vi "Default User.vi"(1 "Account in":string) -> (0 "Account out":string)   [LabVIEW 2019, in "SelfUpdate.lvclass"]
uses:
  SelfUpdate.lvclass
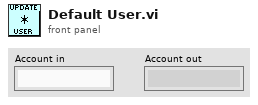
[diagram p1: front panel]
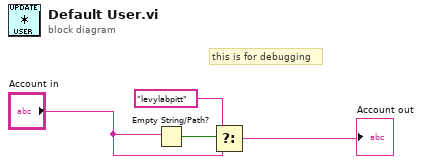
[diagram p0: block diagram]
diagram:
  # "this is for debugging"
  n1 = Empty String/Path?(string/path="Account in") -> (empty?=w1:bool)
  n2 = Select(t="levylabpitt", s=w1, f="Account in") -> (s? t:f=→"Account out":string)
